vi "GammaBurstPhaseTrack.vi"(0 "Input":i32, 5 "Gamma Module\nSettings":T1={"35 Hz"=100, "55 Hz"=100, "75 Hz"=100, "95 Hz"=100, "Min Cycles"=0, "Max Cycles"=0, "Phase Select"=enum."Ascending", "Amplitude"=0} {"Amplitude" scale=0.0..10.0; "95 Hz" scale=0.0..200.0; "75 Hz" scale=0.0..200.0; "55 Hz" scale=0.0..200.0; "35 Hz" scale=0.0..200.0}) -> (4 "PeakAmplitude":i32, 8 "Phase Trigger":bool, 10 "Onset Detect":bool, 15 "Offset Detect":bool)   [LabVIEW 2014]
panel:
  # "Cycle Settings"
  # "Gamma Band Equalizer (% gain)"
  # "Trigger Threshold"
types:
  T1 = cluster{"35 Hz":u8, "55 Hz":u8, "75 Hz":u8, "95 Hz":u8, "Min Cycles":u16, "Max Cycles":u16, "Phase Select":enum16{"Ascending", "Descending", "Peak", "Trough", "Random"}, "Amplitude":i32}
  T2 = enum16{"Ascending", "Descending", "Peak", "Trough", "Random"}
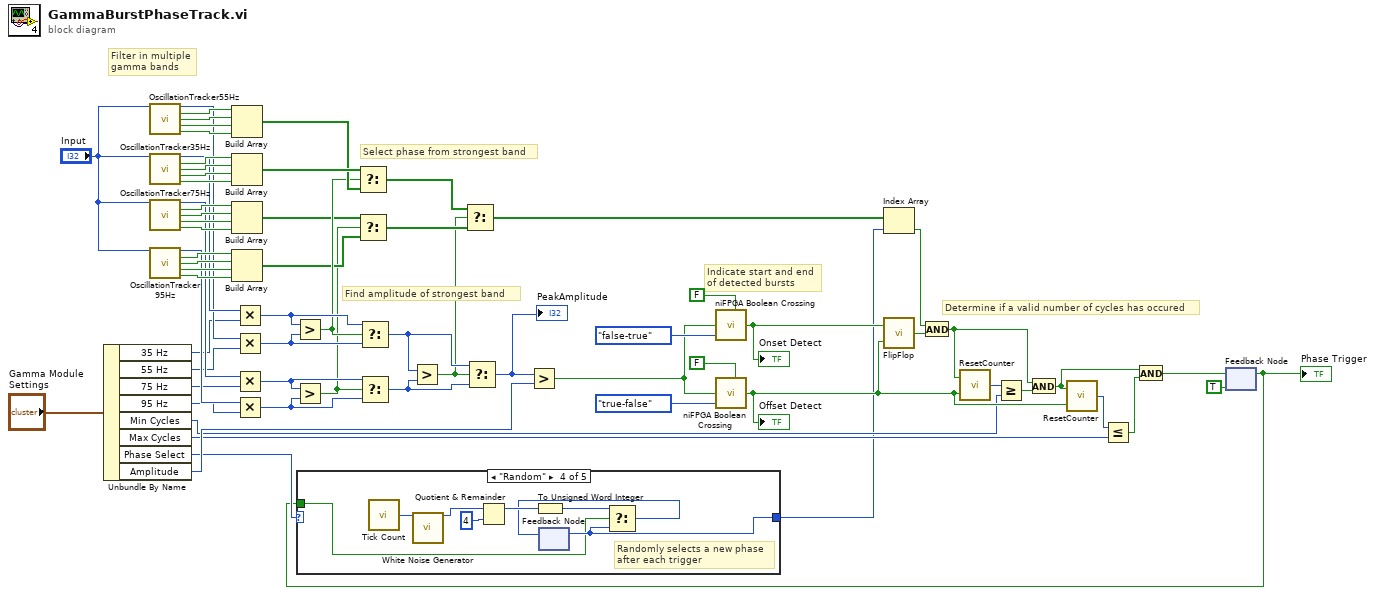
[diagram p0: block diagram]
diagram:
  # "Indicate start and end\nof detected bursts"
  # "Determine if a valid number of cycles has occured"
  # "Filter in multiple\ngamma bands"
  # "Find amplitude of strongest band"
  # "Select phase from strongest band"
  n1 = Unbundle By Name("Gamma Module\nSettings") -> ("35 Hz"=w26:u8, "55 Hz"=w25:u8, "75 Hz"=w24:u8, "95 Hz"=w23:u8, "Min Cycles"=w32:u16, "Max Cycles"=w31:u16, "Phase Select"=w6:T2, "Amplitude"=w33:i32)
  n2 = call "OscillationTracker55Hz.vi"("input data"="Input") -> ("Amplitude"=w29:i32, "Ascending"=w51:bool, "Descending"=w50:bool, "Peak"=w49:bool, "Trough"=w48:bool)  [unwired: 10 in]
  n3 = call "OscillationTracker35Hz.vi"("input data"="Input") -> ("Amplitude"=w30:i32, "Ascending"=w46:bool, "Descending"=w45:bool, "Peak"=w44:bool, "Trough"=w43:bool)  [unwired: 10 in]
  n4 = call "OscillationTracker75Hz.vi"("input data"="Input") -> ("Amplitude"=w28:i32, "Ascending"=w42:bool, "Descending"=w41:bool, "Peak"=w40:bool, "Trough"=w39:bool)  [unwired: 10 in]
  n5 = call "OscillationTracker95Hz.vi"("input data"="Input") -> ("Amplitude"=w27:i32, "Ascending"=w38:bool, "Descending"=w37:bool, "Peak"=w36:bool, "Trough"=w35:bool)  [unwired: 10 in]
  n6 = Build Array(w51, w50, w49, w48) -> (w15:bool[])
  n7 = Build Array(w46, w45, w44, w43) -> (w16:bool[])
  n8 = Build Array(w42, w41, w40, w39) -> (w13:bool[])
  n9 = Build Array(w38, w37, w36, w35) -> (w12:bool[])
  n10 = Multiply(x=w30, y=w26) -> (x*y=w22:i32)
  n11 = Multiply(x=w29, y=w25) -> (x*y=w21:i32)
  n12 = Multiply(x=w28, y=w24) -> (x*y=w20:i32)
  n13 = Multiply(x=w27, y=w23) -> (x*y=w19:i32)
  n14 = Greater?(x=w22, y=w21) -> (0:w14:bool)
  n15 = Greater?(x=w20, y=w19) -> (0:w11:bool)
  n16 = Select(t=w16, s=w14, f=w15) -> (s? t:f=w10:bool[])
  n17 = Select(t=w13, s=w11, f=w12) -> (s? t:f=w9:bool[])
  n18 = Select(t=w22, s=w14, f=w21) -> (s? t:f=w18:i32)
  n19 = Select(t=w20, s=w11, f=w19) -> (s? t:f=w17:i32)
  n20 = Greater?(x=w18, y=w17) -> (0:w8:bool)
  n21 = Select(t=w10, s=w8, f=w9) -> (s? t:f=w7:bool[])
  n22 = Select(t=w18, s=w8, f=w17) -> (s? t:f=w1:i32)
  "PeakAmplitude" <- w1
  n23 = Greater?(x=w1, y=w33) -> (0:w52:bool)
  n24 = call <vilib>:"niFPGA Boolean Crossing.vi"("input"=w52, "direction"=enum8{"either", "false-true", "true-false"}."false-true", "initialize"=FALSE) -> ("crossing"=w63:bool)  [unwired: 6 in]
  "Onset Detect" <- w63
  n25 = call <vilib>:"niFPGA Boolean Crossing.vi"("input"=w52, "direction"=enum8{"either", "false-true", "true-false"}."true-false", "initialize"=FALSE) -> ("crossing"=w56:bool)  [unwired: 6 in]
  "Offset Detect" <- w56
  n26 = call "FlipFlop.vi"("Reset"=w56, "Set"=w63) -> ("Ouput"=w61:bool)
  n27 = feedback #1(TRUE) -> (w3:bool)
  "Phase Trigger" <- w3
  n28 = case shown="\"Random\"" w6 {
    selector: w6 -> [w67 w68 w69 _ w78]
    tunnel: [w67 w68 w69 w71 w78] -> w5
    tunnel: w3 -> [_ _ _ w70 _]
    frame "Ascending", Default {
    }
    frame "Peak" {
    }
    frame "Trough" {
    }
    frame "Random" {
      # "Randomly selects a new phase\nafter each trigger"
      n29 = call "Tick Count"() -> ("Tick Count(Ticks)"=w77:u32)
      n30 = call "White Noise Generator"("seed"=w77) -> ("white noise out"=w76:i16)  [unwired: 14 in]
      n31 = Quotient & Remainder(x=w76, y=i16 4) -> (x-y*floor(x/y)=w74:i16)  [unwired: 1 out]
      n32 = To Unsigned Word Integer(number=w74) -> (unsigned 16bit integer=w73:u16)
      n33 = feedback #2() -> (w71:u16)  [unwired: 1 in]
      n34 = Select(t=w73, s=w70, f=w71) -> (s? t:f=w72:u16)
      n35 = feedback-in #2(w72) -> ()
    }
    frame "Descending" {
    }
  }
  n36 = Index Array(array=w7, index=w5) -> (element=w59:bool)
  n37 = And(x=w59, y=w61) -> (x .and. y?=w60:bool)
  n38 = call "ResetCounter.vi"("Reset"=w56, "Increment"=w60) -> ("x+1"=w58:u16)
  n39 = Greater Or Equal?(x=w58, y=w32) -> (x >= y?=w57:bool)
  n40 = And(x=w60, y=w57) -> (x .and. y?=w53:bool)
  n41 = call "ResetCounter.vi"("Reset"=w56, "Increment"=w53) -> ("x+1"=w55:u16)
  n42 = Less Or Equal?(x=w55, y=w31) -> (x <= y?=w54:bool)
  n43 = And(x=w53, y=w54) -> (x .and. y?=w4:bool)
  n44 = feedback-in #1(w4) -> ()
